vi "ChangeToStaveCoordinateFrame (SubVI).vi"(0 "Array (image frame, specified units)":dbl[][](array[numeric]), 1 "Image Origin in XYZ Stage Coords [mm]":dbl[](array[numeric]), 2 "Units":T1(ring), 3 "Pixel resolution":dbl=3.5) -> (5 "Array (stage frame, mm)":dbl[][](array[numeric]))   [LabVIEW 2016]
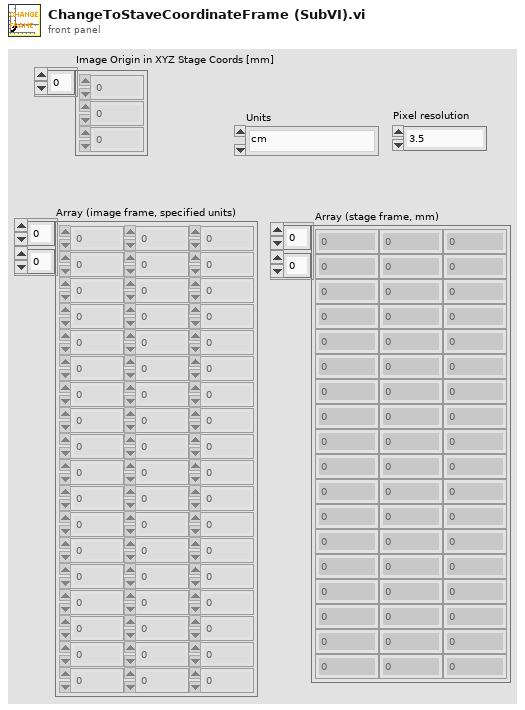
[diagram p1: front panel]
types:
  T1 = enum16{"cm", "mm", "pixels [mm/pix]", "pixels [um/pix]"}
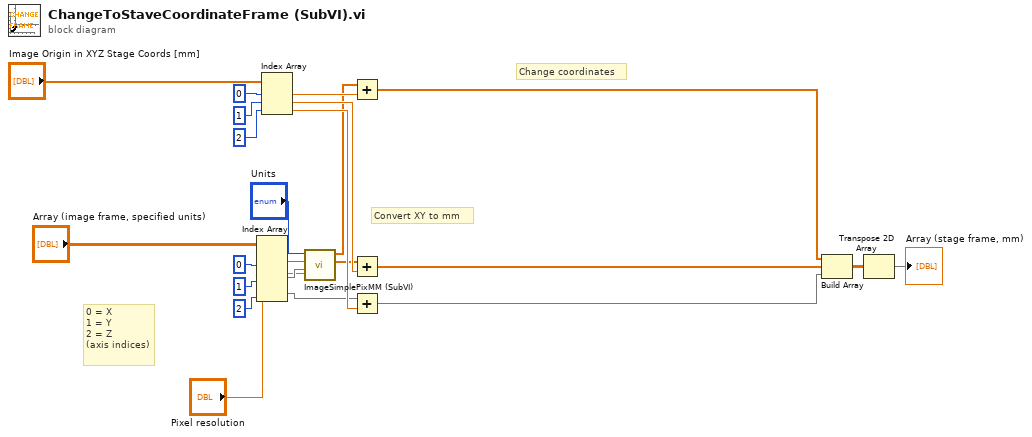
[diagram p0: block diagram]
diagram:
  # "Convert XY to mm"
  # "Change coordinates"
  # "0 = X\n1 = Y\n2 = Z\n(axis indices)"
  n1 = Index Array(array="Array (image frame, specified units)", index (col) #1=0 ("index (row)"), index (col) #2=1 ("index (row)"), index (col) #3=2 ("index (row)")) -> (element #1=w10:dbl[], element #2=w9:dbl[], element #3=w6:dbl[])  [unwired: 3 in]
  n2 = Index Array(array="Image Origin in XYZ Stage Coords [mm]", index #1=0 ("index"), index #2=1 ("index (row)"), index #3=2 ("index (row)")) -> (element #1=w19:dbl, element #2=w15:dbl, element #3=w14:dbl)
  n3 = call "ImageSimplePixMM (SubVI).vi"(6:"Pixel resolution", "Pixel resolution"=w9, "Y Array (image frame, pixels)"=w10, "X Array (image frame,pixels)"="Units") -> ("Y Array (image frame, specified units)"=w7:dbl[], "X Array (image frame, specified units)"=w8:dbl[])  [unwired: 6 in]
  n4 = Add(x=w8, y=w19) -> (x+y=w13:dbl[])
  n5 = Add(x=w7, y=w15) -> (x+y=w12:dbl[])
  n6 = Add(x=w6, y=w14) -> (x+y=w11:dbl[])
  n7 = Build Array(w13, w12, w11) -> (w4:dbl[][])
  n8 = Transpose 2D Array(2D array=w4) -> (transposed array=→"Array (stage frame, mm)":dbl[][])
